vi "Simple Gain Tool .vi"() -> ()   [LabVIEW 2018]
uses:
  <vilib>/addons/control/pid/autopid.llb/PID autotuning parameters (FO).ctl
  <vilib>/DAQmx/write.llb/DAQmx Write (Analog DBL 1Chan 1Samp).vi
  <vilib>/DAQmx/read.llb/DAQmx Read (Analog DBL 1Chan 1Samp).vi
  <vilib>/DAQmx/create/channels.llb/DAQmx Create Channel (AI-Voltage-Basic).vi
  <vilib>/DAQmx/miscellaneous.llb/DAQmx Fill In Error Info.vi
  <vilib>/addons/control/pid/pid.llb/PID Gain Schedule (DBL).vi
  <vilib>/addons/control/pid/pid.llb/PID Advanced (DBL).vi
  <vilib>/addons/control/pid/NI_PID_pid.lvlib
  <vilib>/ptbypt/NI_PtbyPt.lvlib
  <vilib>/addons/control/pid/NI_PID_autopid.lvlib
panel:
  in  "Scaled MV 2":dbl(slide) scale=0.0..2000.0
  out "tuning completed?":bool
  in  "autotuning parameters":T1={"type of controller"=2, "time constant factor"=2.0, "step amplitude"=1.0} {"step amplitude" format="%.2f"; "type of controller" items=["P", "PI", "PID"]}
  out "Scaled MV":dbl(slide) scale=0.0..2000.0
  in  "Target Pressure(in Torr)":dbl
  out "Pressure Readout  (in Torr)":dbl(slide) scale=0.0..1000.0
  out "Pressure (in torr)":dbl
  in  "Sampling Time dt (s)":dbl=0.05 min=0.001 step=0.01 format="%#.3p"
  in  "Stop":bool
  out "SP and PV":cluster{"initial PV":dbl, "SP1:":dbl}(graph)={"initial PV"=50.98160323470328, "SP1:"=50.98039215686275}
  out "PID Gains":T2={"proportional gain (Kc)"=6.925505792902687, "integral time (Ti, min)"=0.004930412653813362, "derivative time (Td, min)"=0.0} {"derivative time (Td, min)" format="%#.6g"; "integral time (Ti, min)" format="%#.6g"; "proportional gain (Kc)" format="%#.6g"}
  in  "Autotune":bool
  in  "Replace gains":bool
  out "MV":dbl(graph)
  out "tuned PID gains":T2={"proportional gain (Kc)"=1.9838195929127882, "integral time (Ti, min)"=0.01995856284686879, "derivative time (Td, min)"=0.0} {"derivative time (Td, min)" format="%#.6g"; "integral time (Ti, min)" format="%#.6g"; "proportional gain (Kc)" format="%#.6g"}
  in  "Reinitialize":bool
  in  "Automatic":bool=TRUE
  in  "alpha":dbl=nan format="%.2f"
  in  "PID gain schedule":T3(array[cluster])=[{"PID gains"={"Kc"=7.0, "Ti"=0.001, "Td"=0.0}, "max value"=0.0}] {"max value" format="%.2f"; "PID gains"."Td" format="%#.3g"; "PID gains"."Ti" format="%#.3g"; "PID gains"."Kc" format="%#.3g"}
  in  "Insert gains":bool
  out "Gain Scheduling":i32
  # "Gain Scheduling"
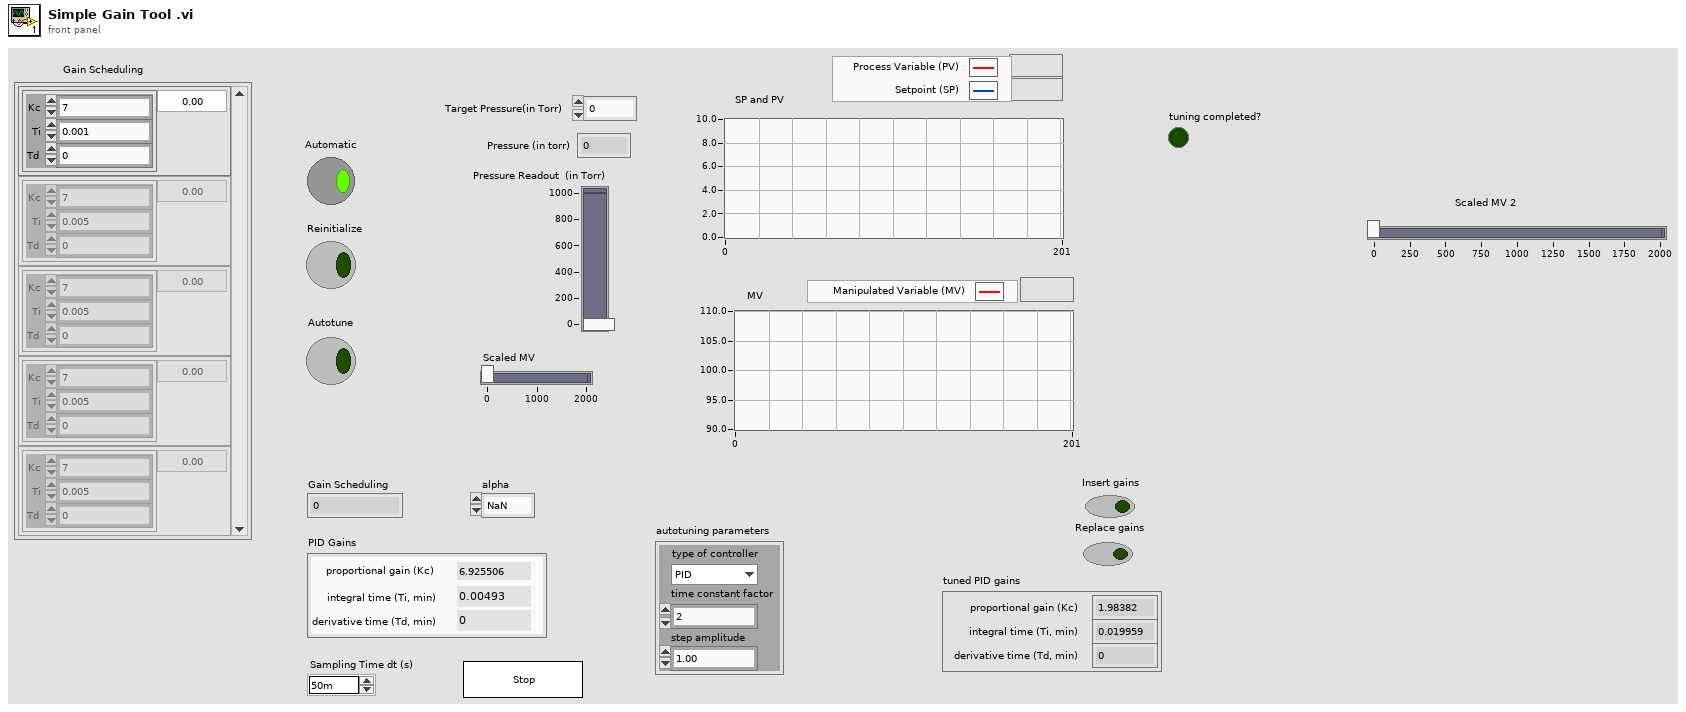
[diagram p1: front panel]
types:
  T1 = typedef "NI_PID_autopid.lvlib/PID autotuning parameters (FO).ctl" = cluster{"type of controller":u16, "time constant factor":dbl, "step amplitude":dbl}
  T2 = cluster{"proportional gain (Kc)":dbl, "integral time (Ti, min)":dbl, "derivative time (Td, min)":dbl}
  T3 = cluster{"PID gains":cluster{"Kc":dbl, "Ti":dbl, "Td":dbl}, "max value":dbl}[]
  T4 = cluster{"process gain":dbl, "time constant (s)":dbl, "delay time (s)":dbl}
  T5 = cluster{"plant parameters out":cluster{"process gain":dbl, "time constant (s)":dbl, "delay time (s)":dbl}, "Target Pressure(in Torr)":dbl}
  T6 = cluster{"PID gains":cluster{"Kc":dbl, "Ti":dbl, "Td":dbl}, "max value":dbl}
  T7 = cluster{"plant parameters out":cluster{"process gain":dbl, "time constant (s)":dbl, "delay time (s)":dbl}, "max value":dbl}
  T8 = cluster{"Pressure Readout  (in Torr)":dbl, "Target Pressure(in Torr)":dbl}
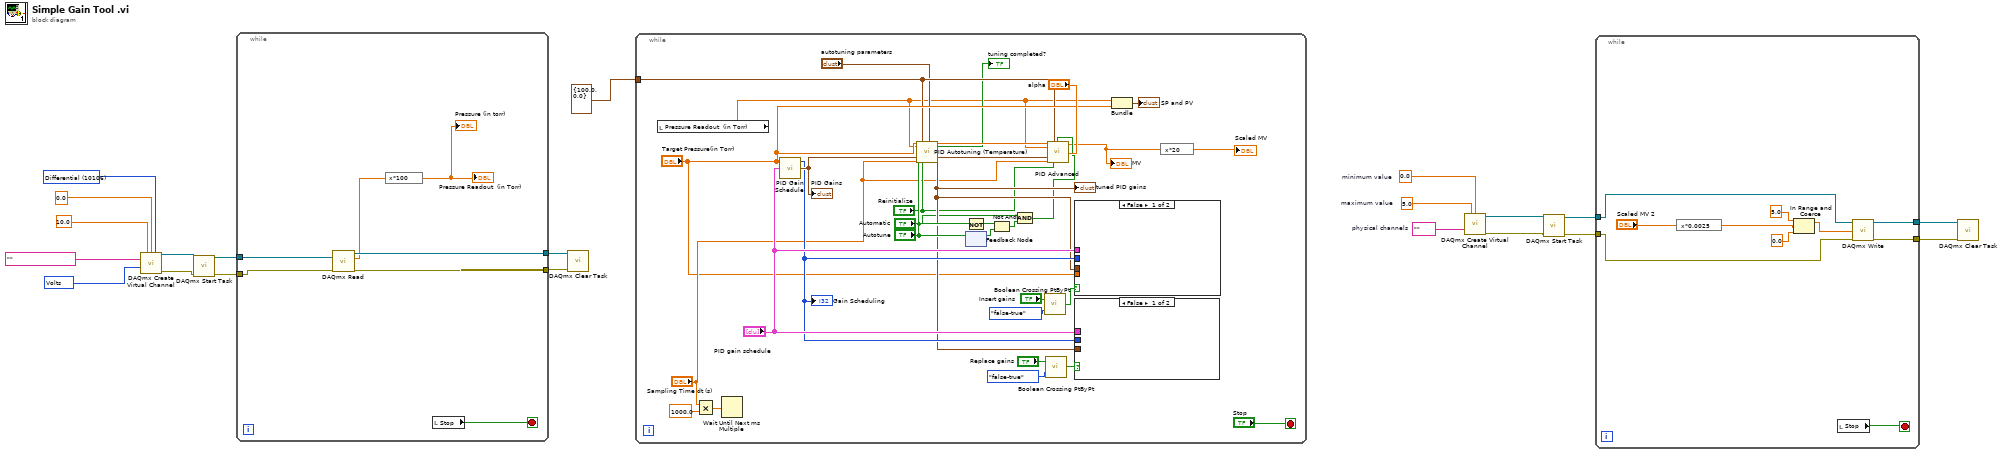
[diagram p0: block diagram]
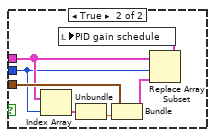
[diagram p2: hidden frame]
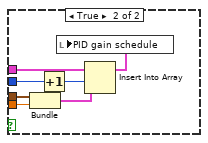
[diagram p3: hidden frame]
diagram:
  w3 = tag ""  # physical channels
  w4 = 0.0  # minimum value
  w5 = 5.0  # maximum value
  w11 = 10348 items=["Volts"=10348, "From Custom Scale"=10065] ("units")
  w13 = 10106 items=["Default"=-1, "RSE"=10083, "NRSE"=10078, "Differential"=10106, "Pseudodifferential"=12529] ("input terminal configuration")
  n1 = call-poly <vilib>:"DAQmx Create Virtual Channel.vi"("maximum value"=10.0, "minimum value"=0.0, "input terminal configuration"=w13, "physical channels"=tag "", "units"=w11) -> ("task out"=w21:refnum<k21>, "error out"=w20:errorcluster)  [unwired: 9 in]
  n2 = call <vilib>:"DAQmx Start Task.vi"("task/channels in"=w21, "error in"=w20) -> ("task out"=w19:refnum<k21>, "error out"=w17:errorcluster)  [unwired: 12 in]
  n3 = while {
    tunnel: w19 -> [w28]
    tunnel: [w27] -> w18
    tunnel: w17 -> [w26]
    tunnel: [w25] -> w16
    stop <- w22 stop-if-true
    n4 = call-poly <vilib>:"DAQmx Read.vi"("task/channels in"=w28, "error in"=w26) -> ("task out"=w27:refnum<k21>, "data"=w24:dbl, "error out"=w25:errorcluster)  [unwired: 11 in]
    n5 = expression code="x*100"(w24) -> (→"Pressure Readout  (in Torr)" →"Pressure (in torr)":dbl)
    n6 = local read "Stop"() -> (w22:bool)
  }
  n7 = call <vilib>:"DAQmx Clear Task.vi"("task in"=w18, "error in"=w16) -> ()  [unwired: 13 in, 1 out]
  n8 = while {
    tunnel: cluster{"output high":dbl, "output low":dbl} {"output high"=100.0, "output low"=0.0} ("output range") -> [w32]
    stop <- "Stop" stop-if-true
    n9 = local read "Pressure Readout  (in Torr)"() -> (w29:dbl)
    n10 = Multiply(x="Sampling Time dt (s)", y=1000.0) -> (x*y=w38:dbl)
    n11 = Wait Until Next ms Multiple(millisecond multiple=w38) -> ()  [unwired: 1 out]
    n12 = call-poly <vilib>:"PID Gain Schedule.vi"("PID gain schedule"="PID gain schedule", "gain scheduling value"="Target Pressure(in Torr)") -> ("PID gains out"=w51:T2, "index out"=w46:i32)  [unwired: 2 in]
    "PID Gains" <- w51
    "Gain Scheduling" <- w46
    n13 = call <vilib>:"PID Autotuning (Temperature).vi"("desired temperature"="Target Pressure(in Torr)", "measured temperature"=w29, "autotune? (F)"="Autotune", "PID gains in"=w51, "dt (s)"="Sampling Time dt (s)", "output range"=w32, "reinitialize? (F)"="Reinitialize", "autotuning parameters"="autotuning parameters") -> ("output"=w59:dbl, "tuning completed?"=→"tuning completed?":bool, "plant parameters out"=w45:T4, "PID gains out"=w58:T2)  [unwired: 8 in]
    "tuned PID gains" <- w45
    n14 = feedback #1() -> (w57:bool)  [unwired: 1 in]
    n15 = feedback-in #1("Autotune") -> ()
    n16 = Not(x="Autotune") -> (.not. x?=w54:bool)
    n17 = Not And(1:w57, 2:w54) -> (0:w55:bool)
    n18 = And(x="Automatic", y=w55) -> (x .and. y?=w42:bool)
    n19 = call <vilib>:"Boolean Crossing PtByPt.vi"("direction"=enum16{"either", "false-true", "true-false"}."false-true", "input"="Insert gains") -> ("crossing"=w52:bool)  [unwired: 1 in]
    n20 = call <vilib>:"Boolean Crossing PtByPt.vi"("direction"=enum16{"either", "false-true", "true-false"}."false-true", "input"="Replace gains") -> ("crossing"=w48:bool)  [unwired: 1 in]
    n21 = call-poly <vilib>:"PID Advanced.vi"("setpoint"=w59, "output range"=w32, "auto? (T)"=w42, "process variable"=w29, "alpha"="alpha", "PID gains"=w58, "dt (s)"="Sampling Time dt (s)", "reinitialize? (F)"="Reinitialize") -> ("output"=w34:dbl)  [unwired: 6 in, 1 out]
    "MV" <- w34
    n22 = case shown="False" w52 {
      tunnel: w45 -> [_ w74]
      tunnel: "Target Pressure(in Torr)" -> [_ w73]
      tunnel: "PID gain schedule" -> [_ w71]
      tunnel: w46 -> [_ w69]
      frame False {
      }
      frame True {
        n23 = Bundle("plant parameters out"=w74, "Target Pressure(in Torr)"=w73) -> (w72:T5)  [unwired: 1 in]
        n24 = Increment(x=w69) -> (x+1=w68:i32)
        n25 = Insert Into Array(array=w71, index=w68, new element=w72) -> (w70:T3)
        n26 = local write "PID gain schedule"(w70) -> ()
      }
    }
    n27 = case shown="False" w48 {
      tunnel: w45 -> [_ w67]
      tunnel: "PID gain schedule" -> [_ w64]
      tunnel: w46 -> [_ w63]
      frame False {
      }
      frame True {
        n28 = Index Array(array=w64, index=w63) -> (element=w62:T6)
        n29 = Unbundle(w62) -> ("max value"=w61:dbl)  [unwired: 1 out]
        n30 = Bundle("plant parameters out"=w67, "max value"=w61) -> (w65:T7)  [unwired: 1 in]
        n31 = Replace Array Subset(array=w64, new element=w65, index=w63) -> (w66:T3)
        n32 = local write "PID gain schedule"(w66) -> ()
      }
    }
    n33 = Bundle("Pressure Readout  (in Torr)"=w29, "Target Pressure(in Torr)"="Target Pressure(in Torr)") -> (→"SP and PV":T8)  [unwired: 1 in]
    n34 = expression code="x*20"(w34) -> (→"Scaled MV":dbl)
  }
  n35 = call-poly <vilib>:"DAQmx Create Virtual Channel.vi"("maximum value"=w5, "minimum value"=w4, "physical channels"=w3) -> ("task out"=w7:refnum<k21>, "error out"=w6:errorcluster)  [unwired: 11 in]
  n36 = call <vilib>:"DAQmx Start Task.vi"("task/channels in"=w7, "error in"=w6) -> ("task out"=w2:refnum<k21>, "error out"=w1:errorcluster)  [unwired: 12 in]
  n37 = while {
    tunnel: [w83] -> w9
    tunnel: [w82] -> w8
    tunnel: w2 -> [w77]
    tunnel: w1 -> [w76]
    stop <- w75 stop-if-true
    n38 = expression code="x*0.0025"("Scaled MV 2") -> (w80:dbl)
    n39 = In Range and Coerce(upper limit=5.0, x=w80, lower limit=0.0) -> (coerced(x)=w81:dbl)  [unwired: 1 out]
    n40 = local read "Stop"() -> (w75:bool)
    n41 = call-poly <vilib>:"DAQmx Write.vi"("task/channels in"=w77, "data"=w81, "error in"=w76) -> ("task out"=w83:refnum<k21>, "error out"=w82:errorcluster)  [unwired: 10 in, 1 out]
  }
  n42 = call <vilib>:"DAQmx Clear Task.vi"("task in"=w9, "error in"=w8) -> ()  [unwired: 13 in, 1 out]
